vi "20220124-vision.vi"() -> ()   [LabVIEW 2019]
panel:
  in  "Stop (F)":bool=TRUE
  out "Array 4":u32[][](array[colorbox])
  out "Array":dbl[](array[numeric])
  out "Array 2":dbl[](array[numeric])
  out "Image Out":T1(plugin-control)
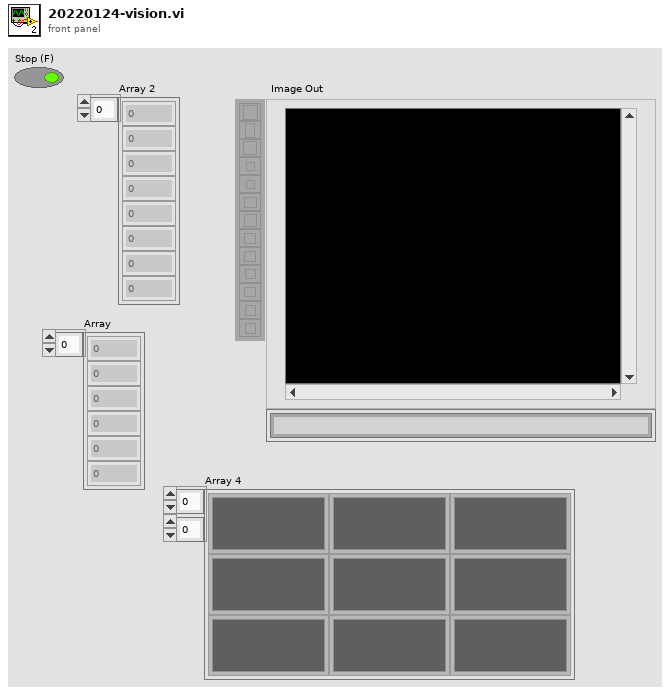
[diagram p1: front panel]
types:
  T1 = typedef "IMAQ Image.ctl" = refnum<image>
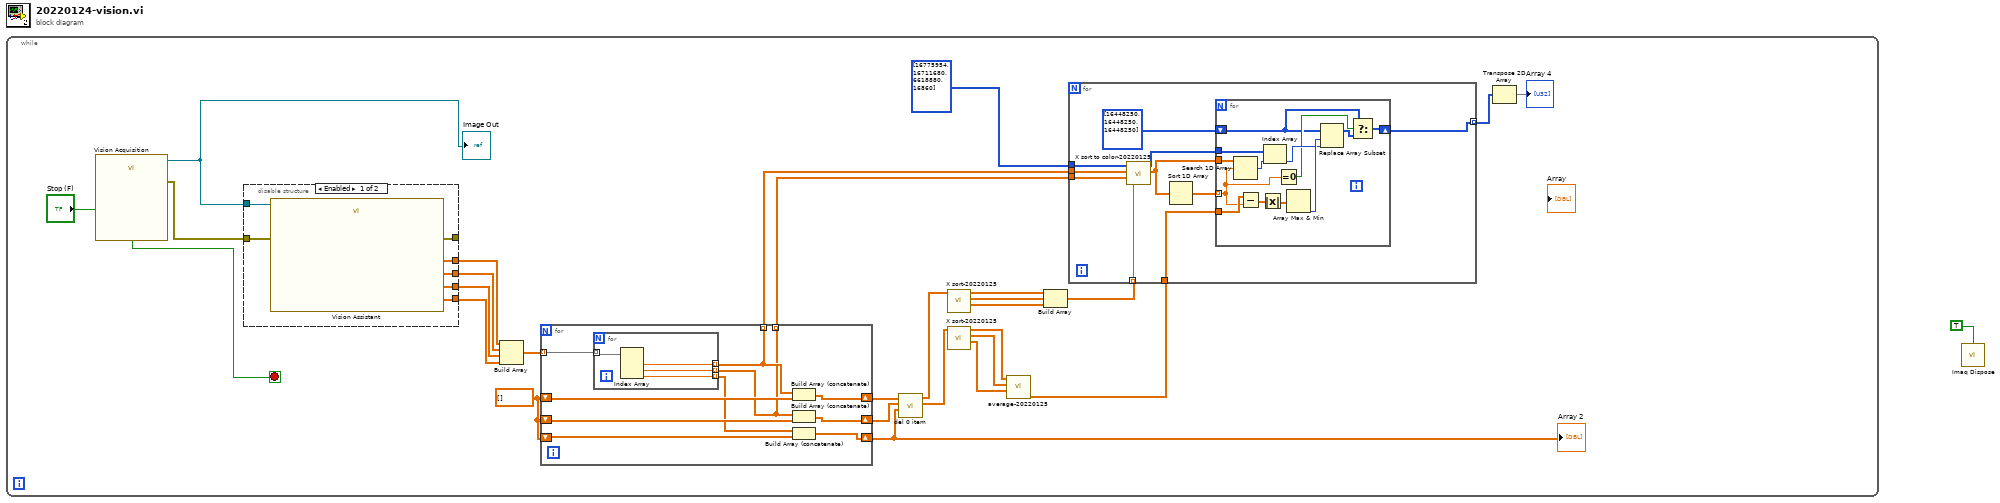
[diagram p0: block diagram]
diagram:
  n1 = while {
    stop <- w27 stop-if-true
    w21 = dbl[] []
    n2 = call "Vision Acquisition"("Stop (F)"="Stop (F)") -> ("Image Out"=w16:T1, "Stopped"=w27:bool, "error out"=w28:errorcluster)  [unwired: 24 in]
    "Image Out" <- w16
    n3 = disable-structure shown="Enabled" {
      disable-tunnel: w28 -> [w59 _]
      disable-tunnel: [w58 _] -> w26
      disable-tunnel: [w57 _] -> w25
      disable-tunnel: [w56 _] -> w24
      disable-tunnel: [w55 _] -> w23
      disable-tunnel: [w54 _] -> _
      disable-tunnel: w16 -> [w53 _]
      frame Enabled {
        n4 = call "Vision Assistant"("Image In"=w53, "error in"=w59) -> ("Particle Measurements (Pixels) (Yellow)"=w58:dbl[][], "Particle Measurements (Pixels) (red)"=w57:dbl[][], "Particle Measurements (Pixels) (green)"=w56:dbl[][], "Particle Measurements (Pixels) (blue)"=w55:dbl[][], "error out"=w54:errorcluster)  [unwired: 20 in, 1 out]
      }
      frame Disabled {
      }
    }
    n5 = Build Array(w26, w25, w24, w23) -> (w22:dbl[][][])
    n6 = for {
      tunnel: w22 -> [w69] mode=indexing
      shift-right: [w67] -> w20
      shift-left: w21 -> [w68]
      shift-right: [w65] -> w19
      shift-left: w21 -> [w66]
      shift-right: [w64] -> w18
      shift-left: w21 -> [w63]
      tunnel: [w61] -> w12 mode=indexing
      tunnel: [w60] -> w11 mode=indexing
      n7 = for {
        tunnel: w69 -> [w73] mode=indexing
        tunnel: [w72] -> w61 mode=indexing
        tunnel: [w71] -> w60 mode=indexing
        tunnel: [w70] -> w62 mode=indexing
        n8 = Index Array(array=w73) -> (element #1=w72:dbl, element #2=w71:dbl, element #3=w70:dbl)  [unwired: 3 in]
      }
      n9 = Build Array (concatenate)(w61, w68) -> (w67:dbl[])
      n10 = Build Array (concatenate)(w60, w66) -> (w65:dbl[])
      n11 = Build Array (concatenate)(w62, w63) -> (w64:dbl[])
    }
    "Array 2" <- w18
    n12 = call "del 0 item.vi"("Array in"=w18, "Y"=w19, "x in"=w20) -> ("Array out"=w17:dbl[], "x out"=w9:dbl[])  [unwired: 7 in]
    n13 = call "X sort-20220125.vi"("x"=w9) -> ("Array 3"=w7:dbl[], "Array 2"=w8:dbl[], "Array"=w6:dbl[])  [unwired: 6 in, 2 out]
    n14 = call "X sort-20220125.vi"("x"=w17) -> ("Array 3"=w13:dbl[], "Array 2"=w14:dbl[], "Array"=w15:dbl[])  [unwired: 6 in, 2 out]
    n15 = call "average-20220125.vi"("3"=w13, "2"=w14, "1"=w15) -> ("Array"=w3:dbl[])  [unwired: 5 in, 3 out]
    n16 = Build Array(w6, w8, w7) -> (w5:dbl[][])
    n17 = for {
      tunnel: w5 -> [w39] mode=indexing
      tunnel: w12 -> [w38]
      tunnel: w11 -> [w37]
      tunnel: u32[] [16775954, 16711680, 6618880, 16860] ("Array") -> [w36]
      tunnel: w3 -> [w31]
      tunnel: [w32] -> w2 mode=indexing
      n18 = call "X sort to color-20220125.vi"("Array 6"=w39, "Array 4"=w37, "Array 5"=w38, "Array in"=w36) -> ("Array 3"=w35:dbl[], "Array out"=w33:u32[])  [unwired: 6 in]
      n19 = Sort 1D Array(array=w35) -> (sorted array=w34:dbl[])
      n20 = for {
        tunnel: w35 -> [w45]
        tunnel: w34 -> [w41] mode=indexing
        tunnel: w33 -> [w48]
        tunnel: w31 -> [w52]
        shift-right: [w44] -> w32
        shift-left: u32[] [16448250, 16448250, 16448250] ("Array") -> [w40]
        n21 = Search 1D Array(1D array=w45, element=w41) -> (index of element=w49:i32)  [unwired: 1 in]
        n22 = Subtract(x=w52, y=w41) -> (x-y=w51:dbl[])
        n23 = Absolute Value(x=w51) -> (abs(x)=w46:dbl[])
        n24 = Index Array(array=w48, index=w49) -> (element=w47:u32)
        n25 = Equal To 0?(x=w41) -> (x = 0?=w42:bool)
        n26 = Array Max & Min(array=w46) -> (min index (indices)=w50:i32)  [unwired: 3 out]
        n27 = Replace Array Subset(array=w40, new element=w47, index=w50) -> (w43:u32[])
        n28 = Select(t=w40, s=w42, f=w43) -> (s? t:f=w44:u32[])
      }
    }
    n29 = Transpose 2D Array(2D array=w2) -> (transposed array=→"Array 4":u32[][])
  }
  n30 = call "Imaq Dispose"("All Images? (No)"=TRUE) -> ()  [unwired: 5 in, 1 out]
